vi "ReadLogNode.vi"(8 "Error In":errorcluster, 11 "Keithley2602 Node In":refnum<k20>) -> (0 "Error Out":errorcluster, 2 "Log Configuration":T1, 3 "Keithley2602 Node Out":refnum<k20>)   [LabVIEW 2012]
uses:
  LogConfiguration.ctl
  LogStartConfiguration.ctl
  LogStartTriggerType.ctl
  LogDigitalIOTriggerEdge.ctl
  LogRolloverConfiguration.ctl
  LogRolloverTriggerType.ctl
  LogStopConfiguration.ctl
  LogStopTriggerType.ctl
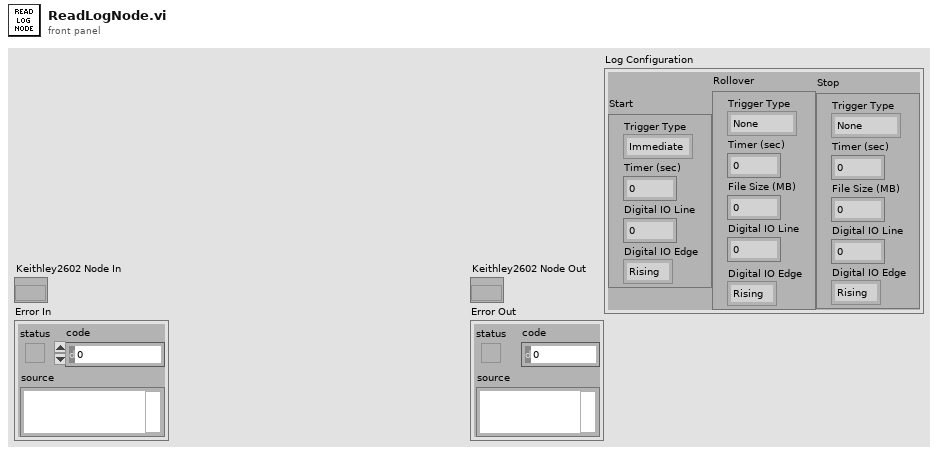
[diagram p1: front panel]
types:
  T1 = typedef "LogConfiguration.ctl" = cluster{"Start":T2, "Rollover":T5, "Stop":T7}
  T2 = typedef "LogStartConfiguration.ctl" = cluster{"Trigger Type":T3, "Timer (sec)":dbl, "Digital IO Line":u8, "Digital IO Edge":T4}
  T3 = typedef "LogStartTriggerType.ctl" = enum16{"Immediate", "User", "Timer", "Digital IO"}
  T4 = typedef "LogDigitalIOTriggerEdge.ctl" = enum16{"Rising", "Falling"}
  T5 = typedef "LogRolloverConfiguration.ctl" = cluster{"Trigger Type":T6, "Timer (sec)":dbl, "File Size (MB)":u32, "Digital IO Line":u8, "Digital IO Edge":T4}
  T6 = typedef "LogRolloverTriggerType.ctl" = enum16{"None", "Timer", "File Size", "Digital IO"}
  T7 = typedef "LogStopConfiguration.ctl" = cluster{"Trigger Type":T8, "Timer (sec)":dbl, "File Size (MB)":u32, "Digital IO Line":u8, "Digital IO Edge":T4}
  T8 = typedef "LogStopTriggerType.ctl" = enum16{"None", "User", "Timer", "File Size", "Digital IO"}
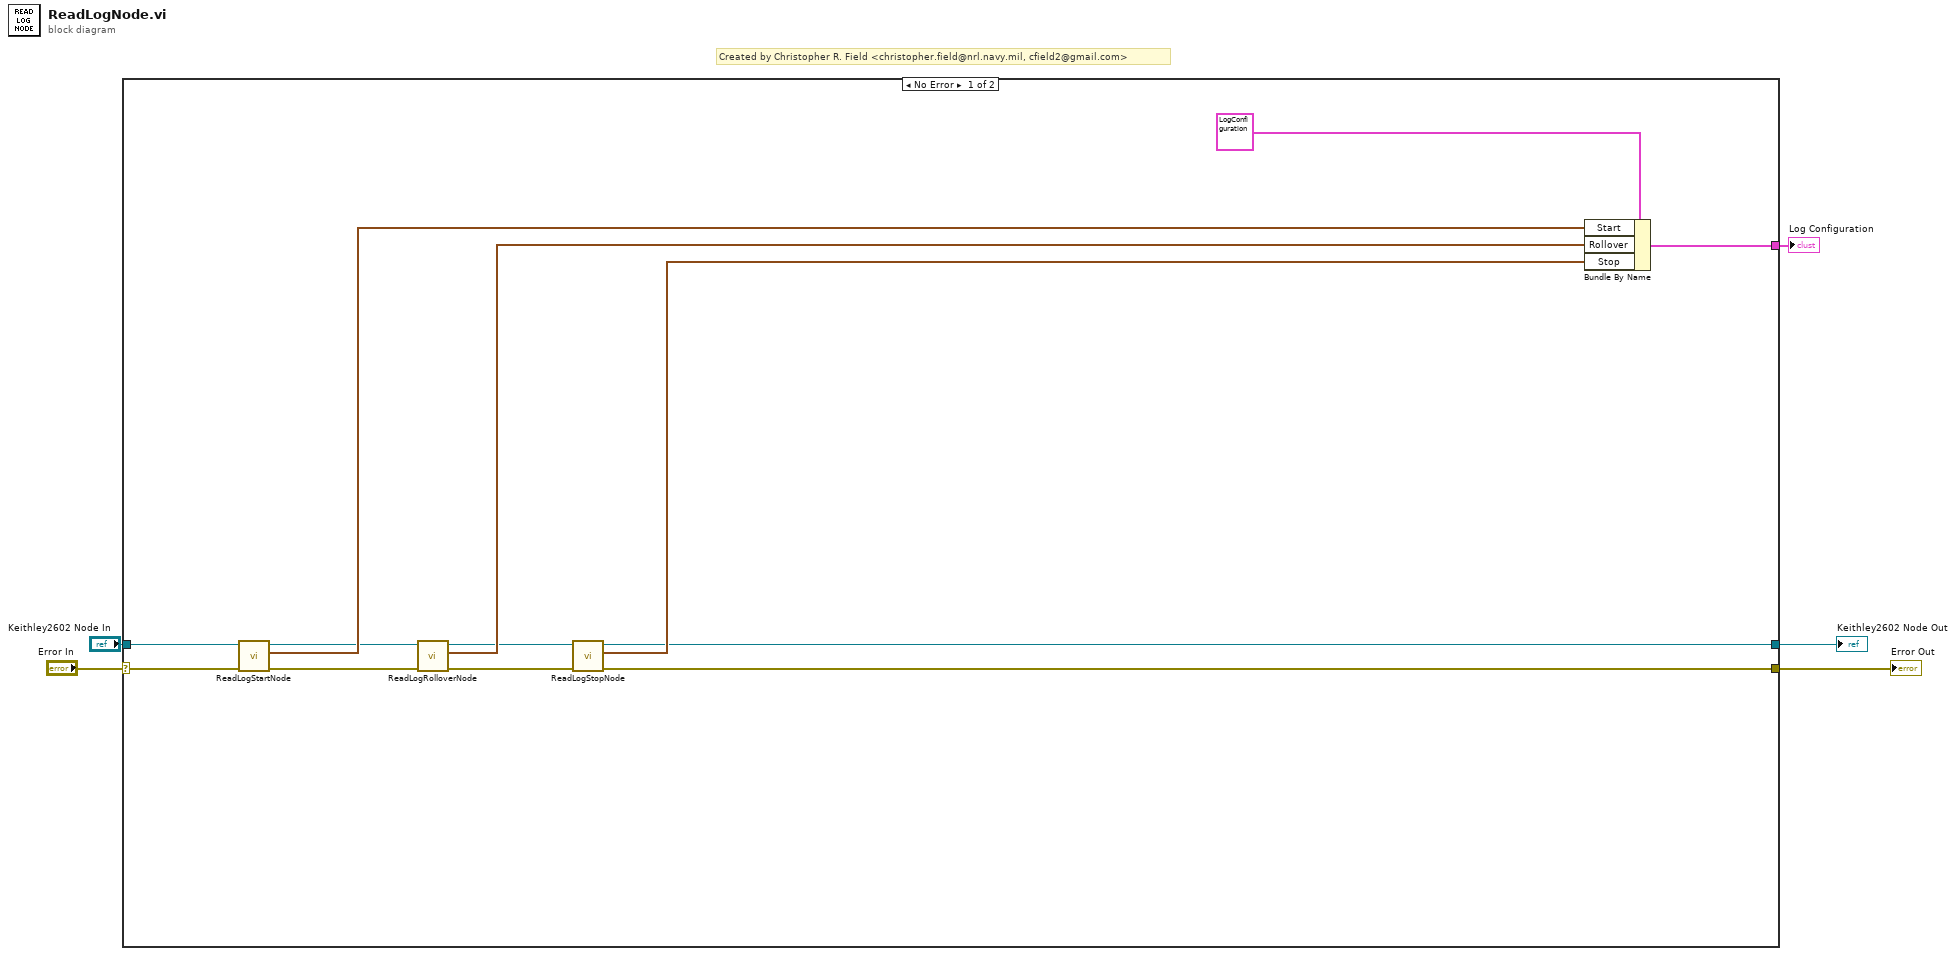
[diagram p0: block diagram]
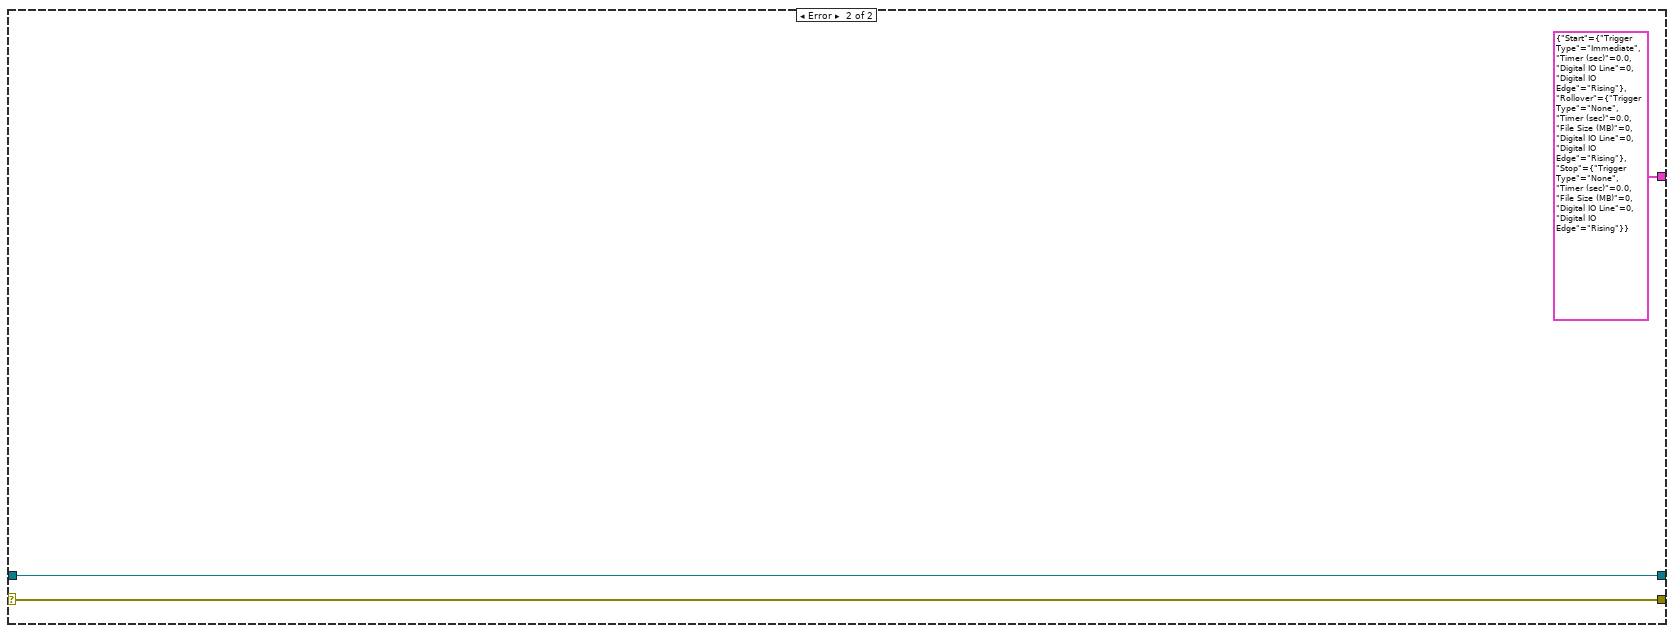
[diagram p2: hidden frame]
diagram:
  # "Created by Christopher R. Field <christopher.field@nrl.navy.mil, cfield2@gmail.com>"
  n1 = case shown="No Error" "Error In" {
    selector: "Error In" -> [w16 w20]
    tunnel: "Keithley2602 Node In" -> [w17 w21]
    tunnel: [w7 w21] -> w3
    tunnel: [w6 w20] -> w2
    tunnel: [w14 T1 {"Start"={"Trigger Type"=enum."Immediate", "Timer (sec)"=0.0, "Digital IO Line"=0, "Digital IO Edge"=enum."Rising"}, "Rollover"={"Trigger Type"=enum."None", "Timer (sec)"=0.0, "File Size (MB)"=0, "Digital IO Line"=0, "Digital IO Edge"=enum."Rising"}, "Stop"={"Trigger Type"=enum."None", "Timer (sec)"=0.0, "File Size (MB)"=0, "Digital IO Line"=0, "Digital IO Edge"=enum."Rising"}} ("Log Configuration")] -> w1
    frame No Error {
      n2 = call "ReadLogStartNode.vi"("Error In"=w16, "Keithley2602 Node In"=w17) -> ("Error Out"=w12:errorcluster, "Log Start Configuration"=w15:T2, "Keithley2602 Node Out"=w13:refnum<k20>)  [unwired: 7 in]
      n3 = call "ReadLogRolloverNode.vi"("Error In"=w12, "Keithley2602 Node In"=w13) -> ("Error Out"=w9:errorcluster, "Log Rollover Configuration"=w11:T5, "Keithley2602 Node Out"=w10:refnum<k20>)  [unwired: 7 in]
      n4 = call "ReadLogStopNode.vi"("Error In"=w9, "Keithley2602 Node In"=w10) -> ("Error Out"=w6:errorcluster, "Log Stop Configuration"=w8:T7, "Keithley2602 Node Out"=w7:refnum<k20>)  [unwired: 7 in]
      n5 = Bundle By Name(cluster=T1 {"Start"={"Trigger Type"=enum."Immediate", "Timer (sec)"=0.0, "Digital IO Line"=0, "Digital IO Edge"=enum."Rising"}, "Rollover"={"Trigger Type"=enum."None", "Timer (sec)"=0.0, "File Size (MB)"=0, "Digital IO Line"=0, "Digital IO Edge"=enum."Rising"}, "Stop"={"Trigger Type"=enum."None", "Timer (sec)"=0.0, "File Size (MB)"=0, "Digital IO Line"=0, "Digital IO Edge"=enum."Rising"}} ("Log Configuration"), "Start"=w15, "Rollover"=w11, "Stop"=w8) -> (w14:T1)
    }
    frame Error {
    }
  }
  "Keithley2602 Node Out" <- w3
  "Error Out" <- w2
  "Log Configuration" <- w1
